vi "csm_lumikki_instron_creep_poller.vi"   [LabVIEW 2009]
doc: "This is the sample data playback waveform and data logging example program. Sample data points are generated using MX Sample Data Array Generator.vi. You will need to replace this VI with your own code. New sample data is sent to the controller each time a status message is recieved from the controller that the next random buffer is running.\nThis program also shows you how to use Active X events. These are used to notify the program when a data buffer is ready for collection and when to load a new buffer of sample data points. Two separate event queues are used: one for data logging and the other for general status, such as when a sample data point buffer can be sent to the controller. Each event handler must run in parallel loops as execution passes to MX Handle Status Change Event.vi and MX Handle Data Ready Event.vi and will not come out of them until an event is received from the console program. When modifiying this example for your own use you may want to setup a third loop to be doing other processing, or you could add code to manipulate the data buffer in the data monitoring loop."
panel:
  # "Axis 1\nAxis 2\nAxis 3\nAxis 4"
  # "Axis 1\nAxis 2\nAxis 3\nAxis 4"
types:
  T1 = cluster{"Name":string, "Type":i32, "SI Full Scale":dbl, "Full Scale":dbl, "Units String":string, "Display Format":string, "Gauge Length":dbl}[][]
  T2 = cluster{"Device ID":i32, "Device Name":string, "Device Type":i32}[]
  T3 = cluster{"Data Sample Format (0)":i8, "Loop code (2)":i8, "Target Amplitude (32767)":i16, "Playback rate":dbl, "Playback Scale":dbl[], "Envelope Ramp Rate":dbl, "Filter Order (0)":i8, "Filter Type (0)":i8, "Filter Bandwidth":dbl}
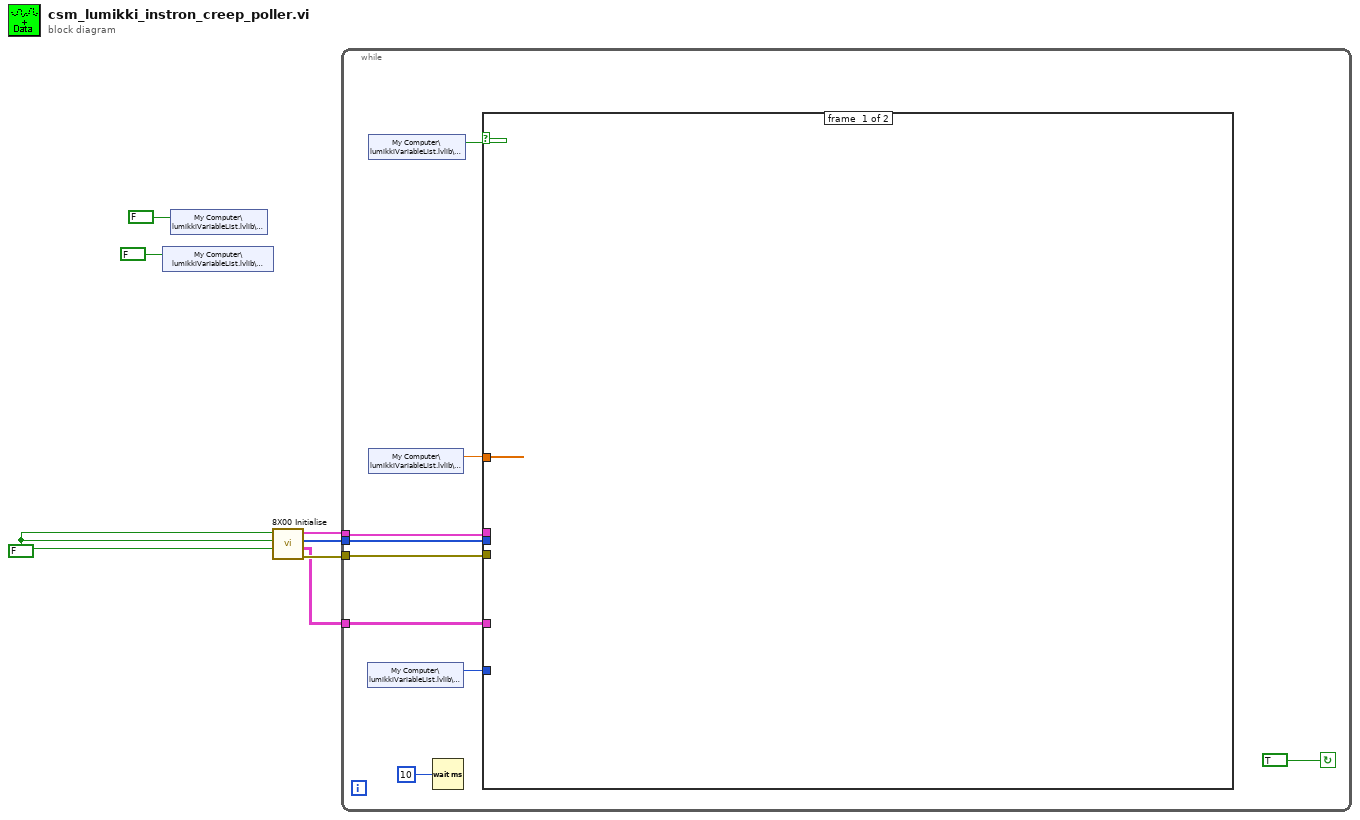
[diagram p0: block diagram]
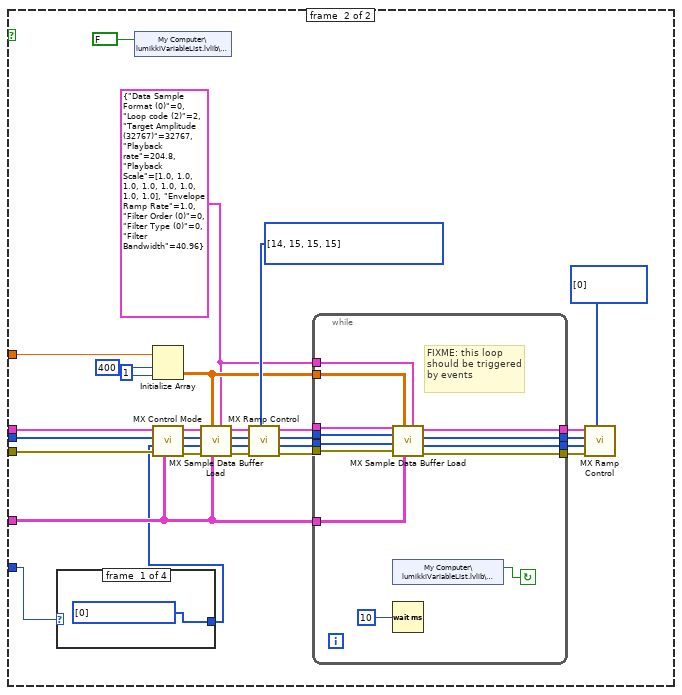
[diagram p2: hidden frame]
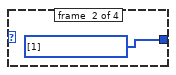
[diagram p3: hidden frame]
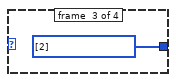
[diagram p4: hidden frame]
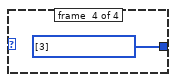
[diagram p5: hidden frame]
diagram:
  w4 = FALSE ("Reset")
  n1 = shared-variable "My Computer\\lumikkiVariableList.lvlib\\creepRunning"(FALSE ("startCreep")) -> ()  [unwired: 1 in, 1 out]
  n2 = shared-variable "My Computer\\lumikkiVariableList.lvlib\\startCreep"(FALSE ("startCreep")) -> ()  [unwired: 1 in, 1 out]
  n3 = call "8X00 Initialise.vi"("Reset?"=w4, "Create DVM? (T)"=w4, "Create Console? (T)"=w4) -> ("error out"=w7:errorcluster, "Channel Data"=w6:T1, "Axis Selector"=w3:i32[], "Axis Information"=w5:T2)  [unwired: 1 in]
  n4 = while {
    tunnel: w6 -> [w16]
    tunnel: w5 -> [w11]
    tunnel: w7 -> [w9]
    tunnel: w3 -> [w10]
    stop <- TRUE continue-if-true
    n5 = shared-variable "My Computer\\lumikkiVariableList.lvlib\\channelInt"() -> (w8:i32)  [unwired: 1 in, 1 out]
    n6 = shared-variable "My Computer\\lumikkiVariableList.lvlib\\startCreep"() -> (w12:bool)  [unwired: 1 in, 1 out]
    n7 = shared-variable "My Computer\\lumikkiVariableList.lvlib\\creepLoad"() -> (w13:dbl)  [unwired: 1 in, 1 out]
    n8 = Wait (ms)(milliseconds to wait=u32 10) -> ()  [unwired: 1 out]
    n9 = case shown="True" w12 {
      tunnel: w16 -> [_ w32]
      tunnel: w13 -> [_ w31]
      tunnel: w11 -> [_ w28]
      tunnel: w10 -> [_ w27]
      tunnel: w9 -> [_ w26]
      tunnel: w8 -> [_ w22]
      frame #0 {
      }
      frame #1 {
        w17 = u16[] [0] items=["Stop", "Start or continue", "Hold", "Continue", "Return ramp to set level at fixed rate", "Reserved", "Reserved", "Start Random without demand hold", "Start Random with demand hold", "Prepare Random Start without demand hold", "Prepare Random Start with demand hold", "Unslave", "Reserved", "Reserved", "Start Sample Data Playback or Resume", "Prepare for Start of Sample Data", "Reserved", "Reserved", "Resume Playback", "Start an electromechanical frame return"] ("Ramp Control")
        w24 = T3 {"Data Sample Format (0)"=0, "Loop code (2)"=2, "Target Amplitude (32767)"=32767, "Playback rate"=204.8, "Playback Scale"=[1.0, 1.0, 1.0, 1.0, 1.0, 1.0, 1.0, 1.0], "Envelope Ramp Rate"=1.0, "Filter Order (0)"=0, "Filter Type (0)"=0, "Filter Bandwidth"=40.96} ("Sample Data Playback Definition")
        w39 = u16[] [14, 15, 15, 15] items=["Stop", "Start or continue", "Hold", "Continue", "Return ramp to set level at fixed rate", "Reserved", "Reserved", "Start Random without demand hold", "Start Random with demand hold", "Prepare Random Start without demand hold", "Prepare Random Start with demand hold", "Unslave", "Reserved", "Reserved", "Start Sample Data Playback or Resume", "Prepare for Start of Sample Data", "Reserved", "Reserved", "Resume Playback"] ("Ramp Control")
        n10 = case shown="1, Default" w22 {
          tunnel: [w47 w48 w49 w50] -> w23
          frame #0 {
            w47 = u16[] [0] items=["Channel 1", "Channel 2", "Channel 3", "Channel 4"] ("Choose channel to apply\nthe setpoint")
          }
          frame #1 {
            w48 = u16[] [1] items=["Channel 1", "Channel 2", "Channel 3", "Channel 4"] ("Choose channel to apply\nthe setpoint")
          }
          frame #2 {
            w49 = u16[] [2] items=["Channel 1", "Channel 2", "Channel 3", "Channel 4"] ("Choose channel to apply\nthe setpoint")
          }
          frame #3 {
            w50 = u16[] [3] items=["Channel 1", "Channel 2", "Channel 3", "Channel 4"] ("Choose channel to apply\nthe setpoint")
          }
        }
        n11 = shared-variable "My Computer\\lumikkiVariableList.lvlib\\startCreep"(FALSE ("startCreep")) -> ()  [unwired: 1 in, 1 out]
        n12 = Initialize Array(w31, 400 ("dimension size"), 1 ("dimension size")) -> (w29:dbl[][])
        n13 = call "MX Control Mode.vi"("Channel Data"=w32, "error in (no error)"=w26, "Control Modes"=w23, "Axis Selector"=w27, "Axis Information"=w28) -> ("error out"=w25:errorcluster, "Control Modes out"=w41:u16[], "Axis Selector out"=w42:i32[], "Axis Information out"=w43:T2)  [unwired: 1 in]
        n14 = call "MX Sample Data Buffer Load.vi"("Sample Data Playback Definition"=w24, "Channel Data"=w32, "Sample Data"=w29, "error in (no error)"=w25, "Channels In"=w41, "Axis Selector In"=w42, "Axis Information In"=w43) -> ("error out"=w44:errorcluster, "Channels Out"=w40:u16[], "Axis Selector Out"=w45:i32[], "Axis Information Out"=w46:T2)  [unwired: 1 in]
        n15 = call "MX Ramp Control.vi"("Ramp Control"=w39, "error in (no error)"=w44, "Channels In"=w40, "Axis Selector In"=w45, "Axis Information In"=w46) -> ("error out"=w34:errorcluster, "Channels Out"=w36:u16[], "Axis Selector Out"=w35:i32[], "Axis Information Out"=w33:T2)  [unwired: 2 in]
        n16 = while {
          tunnel: w33 -> [w63]
          tunnel: w35 -> [w62]
          tunnel: w36 -> [w52]
          tunnel: w34 -> [w61]
          tunnel: [w60] -> w21
          tunnel: [w59] -> w20
          tunnel: [w58] -> w19
          tunnel: [w57] -> w18
          tunnel: w24 -> [w56]
          tunnel: w32 -> [w55]
          tunnel: w29 -> [w53]
          stop <- w54 continue-if-true
          # "FIXME: this loop \nshould be triggered \nby events"
          n17 = call "MX Sample Data Buffer Load.vi"("Sample Data Playback Definition"=w56, "Channel Data"=w55, "Sample Data"=w53, "error in (no error)"=w61, "Channels In"=w52, "Axis Selector In"=w62, "Axis Information In"=w63) -> ("error out"=w57:errorcluster, "Channels Out"=w58:u16[], "Axis Selector Out"=w59:i32[], "Axis Information Out"=w60:T2)  [unwired: 1 in]
          n18 = shared-variable "My Computer\\lumikkiVariableList.lvlib\\creepRunning"() -> (w54:bool)  [unwired: 1 in, 1 out]
          n19 = Wait (ms)(milliseconds to wait=u32 10) -> ()  [unwired: 1 out]
        }
        n20 = call "MX Ramp Control.vi"("Ramp Control"=w17, "error in (no error)"=w18, "Channels In"=w19, "Axis Selector In"=w20, "Axis Information In"=w21) -> ()  [unwired: 2 in, 4 out]
      }
    }
  }
